vi "fileio1.vi"() -> ()   [LabVIEW 2015]
panel:
  in  "file path (use dialog)":path
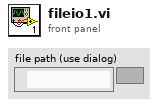
[diagram p1: front panel]
types:
  T1 = enum16{"open", "replace", "create", "open or create", "replace or create", "replace or create with confirmation"}
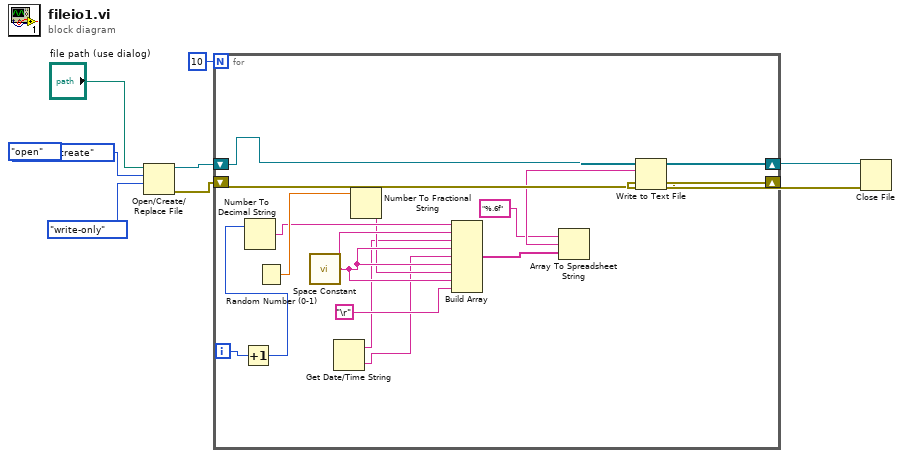
[diagram p0: block diagram]
diagram:
  (unwired) T1."open" ("operation (0:open)")
  n1 = Open/Create/Replace File(file path (use dialog)="file path (use dialog)", operation (0:open)=T1."open or create", access (0:read/write)=enum16{"read/write", "read-only", "write-only"}."write-only") -> (refnum out=w5:refnum<file>, error out=w1:errorcluster)  [unwired: 3 in, 1 out]
  n2 = for {
    N: 10 -> [_]
    shift-right: [w17] -> w4
    shift-left: w5 -> [w18]
    shift-right: [w16] -> w3
    shift-left: w1 -> [w24]
    i -> [w13]
    n3 = Increment(x=w13) -> (x+1=w12:i32)
    n4 = Number To Decimal String(number=w12) -> (decimal integer string=w22:string)  [unwired: 1 in]
    n5 = Random Number (0-1)() -> (number: 0 to 1=w23:dbl)
    n6 = call <vilib>:"Space Constant.vi"() -> ("String"=w15:string)
    n7 = Get Date/Time String() -> (date string=w10:string, time string=w9:string)  [unwired: 3 in]
    n8 = Number To Fractional String(number=w23) -> (F-format string=w11:string)  [unwired: 3 in]
    n9 = Build Array(w22, w15, w10, w15, w9, w15, w11, w15, "\r") -> (w20:string[])
    n10 = Array To Spreadsheet String(array=w20, 3:"%.6f" ("format string")) -> (spreadsheet string=w21:string)  [unwired: 1 in]
    n11 = Write to Text File(file (use dialog)=w18, text=w21, error in=w24) -> (refnum out=w17:refnum<file>, error out=w16:errorcluster)  [unwired: 1 in, 1 out]
  }
  n12 = Close File(refnum=w4, error in=w3) -> ()  [unwired: 2 out]
